vi "ERR HANDLER - Check Error.vi"() -> (1 "ABORT":bool)   [LabVIEW 2013]
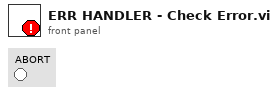
[diagram p1: front panel]
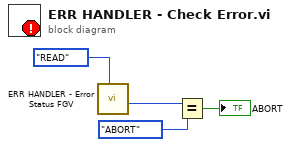
[diagram p0: block diagram]
diagram:
  n1 = call "ERR HANDLER - Error Status FGV.vi"("Method"=enum16{"READ", "WRITE"}."READ") -> ("Abort Program (R)"=w3:enum16{"Not Yet", "ABORT"})  [unwired: 8 in, 2 out]
  n2 = Equal?(x=w3, y=enum16{"Not Yet", "ABORT"}."ABORT") -> (x = y?=→"ABORT":bool)
